vi "Begin.vi"(8 "error in":errorcluster) -> (0 "error out":errorcluster)   [LabVIEW 2023]
doc: "Called before other user functions, this VI can be used to open I/O refnums, load in file data, and do general program initialization. Notice that the <B>error out</B> terminal is simply used for data flow. Wiring it to other structures or subVIs ensures that this VI runs first."
uses:
  <vilib>/Rock Robotics/WPI/DriverStation/WPI_DriverStationRobotMode2.ctl
  <vilib>/Rock Robotics/WPI/Joystick/WPI_JoystickDeviceEnum.ctl
  <vilib>/Rock Robotics/SystemInterfaces/DIO/FPGA_DIOChannel.ctl
  <vilib>/Rock Robotics/WPI/ThirdParty/REV Robotics/REVLib/Typedef/Spark MAX Motor Type.ctl
  <vilib>/Rock Robotics/WPI/ThirdParty/REV Robotics/REVLib/Typedef/Spark MAX Idle Mode.ctl
  <vilib>/Rock Robotics/WPI/ThirdParty/REV Robotics/REVLib/Typedef/Spark MAX Sensor Type.ctl
  MHZLib/Variables and Definitions/Robot Global Data.vi
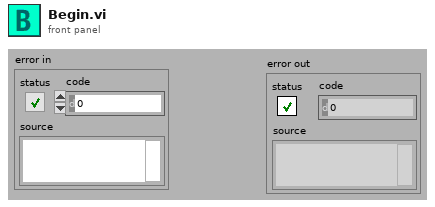
[diagram p1: front panel]
types:
  T1 = cluster{"P Gain":dbl, "I Gain":dbl, "D Gain":dbl, "F Gain":dbl, "I Zone":dbl, "Min Output":dbl, "Max Output":dbl}
  T2 = typedef "FPGA_DIOChannel.ctl" = enum8{"DIO 0", "DIO 1", "DIO 2", "DIO 3", "DIO 4", "DIO 5", "DIO 6", "DIO 7", "DIO 8", "DIO 9", "DIO MXP 0", "DIO MXP 1", "DIO MXP 2", "DIO MXP 3", "DIO MXP 4", "DIO MXP 5", "DIO MXP 6", "DIO MXP 7", "DIO MXP 8", "DIO MXP 9", "DIO MXP 10", "DIO MXP 11", "DIO MXP 12", "DIO MXP 13", "DIO MXP 14", "DIO MXP 15", "SPI Port CS1", "SPI Port CS2", "SPI Port CS3", "SPI Port MISO", "SPI Port MOSI", "Invalid"}
  T3 = typedef "Spark MAX Sensor Type.ctl" = enum16{"No Sensor", "Hall Sensor", "Encoder", "-Not Available-", "Analog", "Alternate Encoder", "Duty Cycle"}
  T4 = typedef "Spark MAX Idle Mode.ctl" = enum16{"Coast", "Brake"}
  T5 = typedef "Spark MAX Motor Type.ctl" = enum16{"Brushed", "Brushless"}
  T6 = typedef "WPI_JoystickDeviceEnum.ctl" = enum16{"USB 0", "USB 1", "USB 2", "USB 3", "USB 4", "USB 5"}
  T7 = cluster{"Drive FL Invert?":bool, "Drive BL Invert?":bool, "Drive FR Invert?":bool, "Drive BR Invert?":bool}
  T8 = cluster{"Drive FL ID":u8, "Drive FR ID":u8, "Drive BL ID":u8, "Drive BR ID":u8}
  T9 = cluster{"Steer FL ID":u8, "Steer FR ID":u8, "Steer BL ID":u8, "Steer BR ID":u8}
  T10 = typedef "WPI_DriverStationRobotMode2.ctl" = enum16{"Autonomous Disabled", "Autonomous Enabled", "Teleop Disabled", "Teleop Enabled", "Disconnected", "Finish", "Test Disabled", "Test Enabled", "Emergency Stopped"}
  T11 = typedef "WPI_JoystickDevRef.ctl" = cluster{"Device":T6}
  T12 = typedef "DeviceReference.ctl" = cluster{"CANbus Name":string, "Device Encoding":u32, "Device Name":string}
  T13 = typedef "WPI_MotorControlDeviceRef.ctl" = cluster{"DeviceStatus":errorcluster, "Type":T14, "PWM":cluster{"PWM Channel":T15, "DeadBand":T16}, "CAN":cluster{"Device Number":u8, "SetOutput VI Ref":variant, "GetOutput VI Ref":variant, "Enable VI Ref":variant, "Disable VI Ref":variant, "Data":variant}, "Invert":bool, "DIO PWM":cluster{"PWM \"Enable\" Channel":T15, "DIOChannel":T2, "PWM Rate":dbl}}
  T14 = typedef "WPI_MotorControlType.ctl" = enum16{"PWM", "CAN", "DIO PWM"}
  T15 = typedef "FPGA_DIOPWMChannel.ctl" = enum8{"PWM 0", "PWM 1", "PWM 2", "PWM 3", "PWM 4", "PWM 5", "PWM 6", "PWM 7", "PWM 8", "PWM 9", "PWM MXP 0", "PWM MXP 1", "PWM MXP 2", "PWM MXP 3", "PWM MXP 4", "PWM MXP 5", "PWM MXP 6", "PWM MXP 7", "PWM MXP 8", "PWM MXP 9", "Invalid"}
  T16 = typedef "WPI_PWMDeadband.ctl" = cluster{"Name":string, "maxPositivePwm":i32, "minPositivePwm":i32, "centerPwm":i32, "maxNegativePwm":i32, "minNegativePwm":i32, "angularRange":u16}
  T17 = typedef "WPI_DigitalInputDevRef.ctl" = cluster{"DevStatus":errorcluster, "DIO Channel":T2}
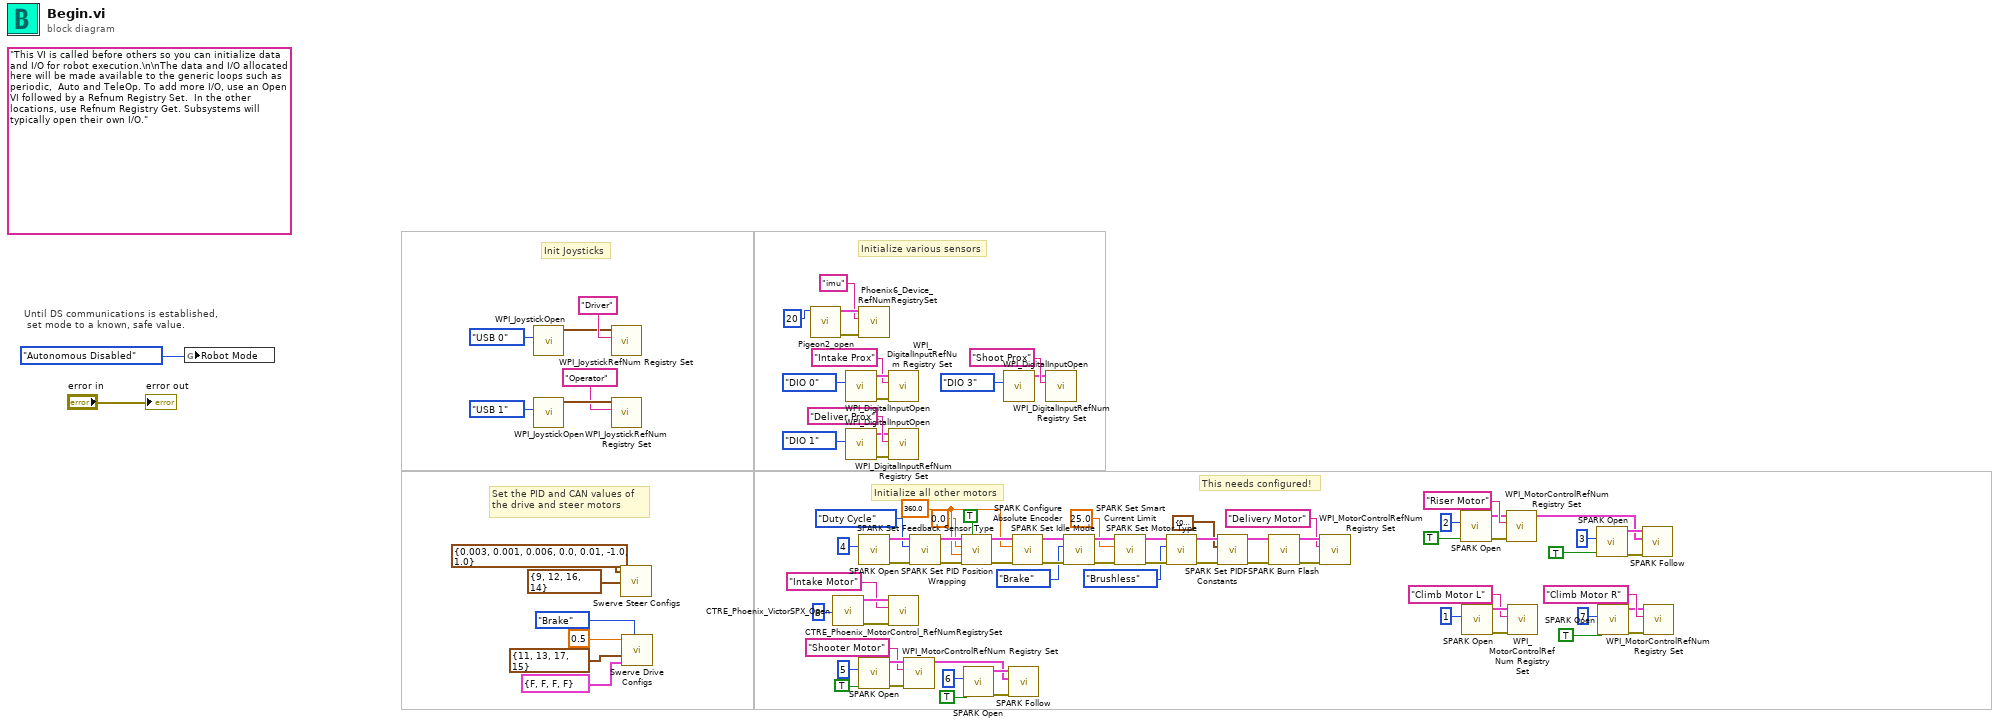
[diagram p0: block diagram]
diagram:
  w37 = 360.0 ("Position Conversion Factor (1)")
  (unwired) "This VI is called before others so you can initialize data and I/O for robot execution.\n\nThe data and I/O allocated here will be made available to the generic loops such as periodic,  Auto and TeleOp. To add more I/O, use an Open VI followed by a Refnum Registry Set.  In the other locations, use Refnum Registry Get. Subsystems will typically open their own I/O."
  # "This needs configured!"
  # "Initialize all other motors"
  # "Init Joysticks"
  # "Initialize various sensors"
  # "Set the PID and CAN values of\nthe drive and steer motors"
  # "Until DS communications is established,\n set mode to a known, safe value."
  n1 = global write "Robot Global Data.vi" "Robot Mode"(WPI_DriverStationRobotMode2."Autonomous Disabled" ("Robot Mode")) -> ()
  n2 = call <vilib>:"WPI_JoystickOpen.vi"("JoystickDevice"=WPI_JoystickDeviceEnum."USB 0") -> ("JoystickDevRef"=w88:T11)  [unwired: 10 in]
  n3 = call <vilib>:"WPI_JoystickOpen.vi"("JoystickDevice"=WPI_JoystickDeviceEnum."USB 1") -> ("JoystickDevRef"=w74:T11)  [unwired: 10 in]
  n4 = call <vilib>:"WPI_JoystickRefNum Registry Set.vi"("refnum name"="Driver", "JoystickDevRef"=w88) -> ()  [unwired: 8 in, 2 out]
  n5 = call <vilib>:"WPI_JoystickRefNum Registry Set.vi"("refnum name"="Operator", "JoystickDevRef"=w74) -> ()  [unwired: 8 in, 2 out]
  n6 = call "Swerve Steer Configs.vi"("Input IDs"=T9 {"Steer FL ID"=9, "Steer FR ID"=12, "Steer BL ID"=16, "Steer BR ID"=14}, "PID Constants"=T1 {"P Gain"=0.003, "I Gain"=0.001, "D Gain"=0.006, "F Gain"=0.0, "I Zone"=0.01, "Min Output"=-1.0, "Max Output"=1.0}) -> ()  [unwired: 2 in]
  n7 = call "Swerve Drive Configs.vi"("Ramp Rate"=sgl 0.5, "Input IDs"=T8 {"Drive FL ID"=11, "Drive FR ID"=13, "Drive BL ID"=17, "Drive BR ID"=15}, "Inversions?"=T7 {"Drive FL Invert?"=FALSE, "Drive BL Invert?"=FALSE, "Drive FR Invert?"=FALSE, "Drive BR Invert?"=FALSE}, "Idle Mode"=Spark_MAX_Idle_Mode."Brake") -> ()  [unwired: 4 in]
  n8 = call <vilib>:"Pigeon2_open.vi"("Device ID"=u8 20 ("Device Number")) -> ("error out"=w78:errorcluster, "DeviceReference 2"=w77:T12)  [unwired: 9 in]
  n9 = call <vilib>:"CTRE_Phoenix_VictorSPX_Open.vi"("Device Number"=u8 8) -> ("error out"=w9:errorcluster, "PhoenixMotorControlDevRef"=w8:T13)  [unwired: 9 in]
  n10 = call <vilib>:"WPI_DigitalInputOpen.vi"("DIO Channel"=FPGA_DIOChannel."DIO 0") -> ("error out"=w72:errorcluster, "DigitalInputDevRef"=w71:T17)  [unwired: 9 in]
  n11 = call <vilib>:"WPI_DigitalInputOpen.vi"("DIO Channel"=FPGA_DIOChannel."DIO 1") -> ("error out"=w67:errorcluster, "DigitalInputDevRef"=w68:T17)  [unwired: 9 in]
  n12 = call <vilib>:"Phoenix6_Device_RefNumRegistrySet.vi"("error in (no error)"=w78, "refnum name"="imu", "DeviceReference"=w77) -> ()  [unwired: 7 in, 2 out]
  n13 = call <vilib>:"SPARK Open.vi"("Device Number"=u8 4) -> ("error out"=w44:errorcluster, "MotorControlDeviceRef"=w45:T13)  [unwired: 9 in]
  n14 = call <vilib>:"SPARK Open.vi"("Invert"=TRUE, "Device Number"=u8 5) -> ("error out"=w32:errorcluster, "MotorControlDeviceRef"=w31:T13)  [unwired: 8 in]
  n15 = call <vilib>:"WPI_DigitalInputRefNum Registry Set.vi"("error in (no error)"=w72, "refnum name"="Intake Prox", "DigitalInputDevRef"=w71) -> ()  [unwired: 7 in, 2 out]
  n16 = call <vilib>:"WPI_DigitalInputRefNum Registry Set.vi"("error in (no error)"=w67, "refnum name"="Deliver Prox", "DigitalInputDevRef"=w68) -> ()  [unwired: 7 in, 2 out]
  n17 = call <vilib>:"CTRE_Phoenix_MotorControl_RefNumRegistrySet.vi"("error in (no error)"=w9, "refnum name"="Intake Motor", "PhoenixMotorControlDevRef"=w8) -> ()  [unwired: 7 in, 2 out]
  n18 = call <vilib>:"WPI_MotorControlRefNum Registry Set.vi"("error in (no error)"=w32, "refnum name"="Shooter Motor", "MotorControlDevRef"=w31) -> ("MotorControlDevRef"=w11:T13)  [unwired: 7 in, 1 out]
  n19 = call <vilib>:"SPARK Set Feedback Sensor Type.vi"("error in (no error)"=w44, "Sensor Type"=Spark_MAX_Sensor_Type."Duty Cycle", "MotorControlDevRef"=w45) -> ("error out"=w54:errorcluster, "MotorControlDeviceRef"=w55:T13)  [unwired: 7 in]
  n20 = call <vilib>:"SPARK Set PID Position Wrapping.vi"("Enable (F)"=TRUE, "error in (no error)"=w54, "Maximum Output (0)"=w37, "Minimum Input (0)"=0.0 ("Position Conversion Factor (1)"), "MotorControlDeviceRef in"=w55) -> ("error out"=w56:errorcluster, "MotorControlDeviceRef out"=w57:T13)  [unwired: 5 in]
  n21 = call <vilib>:"SPARK Open.vi"("Invert"=TRUE, "Device Number"=u8 6) -> ("error out"=w28:errorcluster, "MotorControlDeviceRef"=w29:T13)  [unwired: 8 in]
  n22 = call <vilib>:"WPI_DigitalInputOpen.vi"("DIO Channel"=FPGA_DIOChannel."DIO 3") -> ("DigitalInputDevRef"=w24:T17)  [unwired: 9 in, 1 out]
  n23 = call <vilib>:"SPARK Follow.vi"("error in (no error)"=w28, "Master Controller"=w11, "MotorControlDeviceRef"=w29) -> ()  [unwired: 7 in, 2 out]
  n24 = call <vilib>:"SPARK Configure Absolute Encoder.vi"("error in (no error)"=w56, "Position Conversion Factor (1)"=w37, "MotorControlDeviceRef in"=w57) -> ("error out"=w58:errorcluster, "MotorControlDeviceRef out"=w59:T13)  [unwired: 7 in]
  n25 = call <vilib>:"WPI_DigitalInputRefNum Registry Set.vi"("refnum name"="Shoot Prox", "DigitalInputDevRef"=w24) -> ()  [unwired: 8 in, 2 out]
  n26 = call <vilib>:"SPARK Set Idle Mode.vi"("error in (no error)"=w58, "Idle Mode"=Spark_MAX_Idle_Mode."Brake", "MotorControlDeviceRef in"=w59) -> ("error out"=w51:errorcluster, "MotorControlDeviceRef out"=w50:T13)  [unwired: 7 in]
  n27 = call <vilib>:"SPARK Set Smart Current Limit.vi"("error in (no error)"=w51, "Primay Current Limit (80A)"=25.0, "MotorControlDeviceRef in"=w50) -> ("error out"=w49:errorcluster, "MotorControlDeviceRef out"=w48:T13)  [unwired: 7 in]
  n28 = call <vilib>:"SPARK Set Motor Type.vi"("error in (no error)"=w49, "Motor Type"=Spark_MAX_Motor_Type."Brushless", "MotorControlDevRef"=w48) -> ("error out"=w46:errorcluster, "MotorControlDeviceRef"=w47:T13)  [unwired: 7 in]
  n29 = call <vilib>:"SPARK Set PIDF Constants.vi"("error in"=w46, "PID Constants"=T1 {"P Gain"=0.003, "I Gain"=0.0, "D Gain"=0.006, "F Gain"=0.0, "I Zone"=0.01, "Min Output"=-0.1, "Max Output"=0.1}, "MotorControlDeviceRef"=w47) -> ("error out"=w52:errorcluster, "MotorControlDeviceRef"=w53:T13)  [unwired: 7 in]
  n30 = call <vilib>:"SPARK Burn Flash.vi"("error in"=w52, "MotorControlDeviceRef"=w53) -> ("error out"=w42:errorcluster, "MotorControlDeviceRef"=w43:T13)  [unwired: 8 in]
  n31 = call <vilib>:"WPI_MotorControlRefNum Registry Set.vi"("error in (no error)"=w42, "refnum name"="Delivery Motor", "MotorControlDevRef"=w43) -> ()  [unwired: 7 in, 2 out]
  n32 = call <vilib>:"SPARK Open.vi"("Invert"=TRUE, "Device Number"=u8 2) -> ("error out"=w62:errorcluster, "MotorControlDeviceRef"=w63:T13)  [unwired: 8 in]
  n33 = call <vilib>:"SPARK Open.vi"("Device Number"=u8 1) -> ("error out"=w14:errorcluster, "MotorControlDeviceRef"=w13:T13)  [unwired: 9 in]
  n34 = call <vilib>:"WPI_MotorControlRefNum Registry Set.vi"("error in (no error)"=w62, "refnum name"="Riser Motor", "MotorControlDevRef"=w63) -> ("MotorControlDevRef"=w10:T13)  [unwired: 7 in, 1 out]
  n35 = call <vilib>:"WPI_MotorControlRefNum Registry Set.vi"("error in (no error)"=w14, "refnum name"="Climb Motor L", "MotorControlDevRef"=w13) -> ()  [unwired: 7 in, 2 out]
  n36 = call <vilib>:"SPARK Open.vi"("Invert"=TRUE, "Device Number"=u8 3) -> ("error out"=w21:errorcluster, "MotorControlDeviceRef"=w20:T13)  [unwired: 8 in]
  n37 = call <vilib>:"SPARK Open.vi"("Invert"=TRUE, "Device Number"=u8 7) -> ("error out"=w17:errorcluster, "MotorControlDeviceRef"=w18:T13)  [unwired: 8 in]
  n38 = call <vilib>:"SPARK Follow.vi"("error in (no error)"=w21, "Master Controller"=w10, "MotorControlDeviceRef"=w20) -> ()  [unwired: 7 in, 2 out]
  n39 = call <vilib>:"WPI_MotorControlRefNum Registry Set.vi"("error in (no error)"=w17, "refnum name"="Climb Motor R", "MotorControlDevRef"=w18) -> ()  [unwired: 7 in, 2 out]
  "error out" <- "error in"
